vi "Lock Controls.vi"(8 "error in (no error)":errorcluster, 10 "Lock Controls?":bool, 11 "PXIe5105 in":refnum<class "PXIe5105.lvclass">) -> (0 "error out":errorcluster, 3 "PXIe5105 out":refnum<class "PXIe5105.lvclass">)   [LabVIEW 2018, in "PXIe5105.lvlib" / "PXIe5105.lvclass"]
doc: "This override method is used to lock/unlock user access to the oscilloscope front panel controls."
uses:
  PXIe5105.lvclass
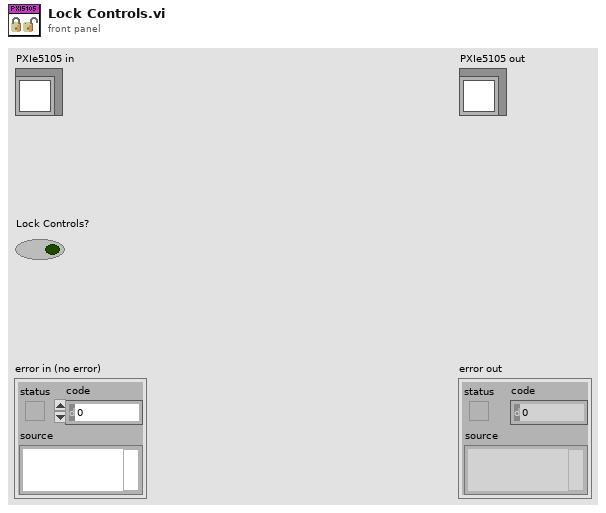
[diagram p1: front panel]
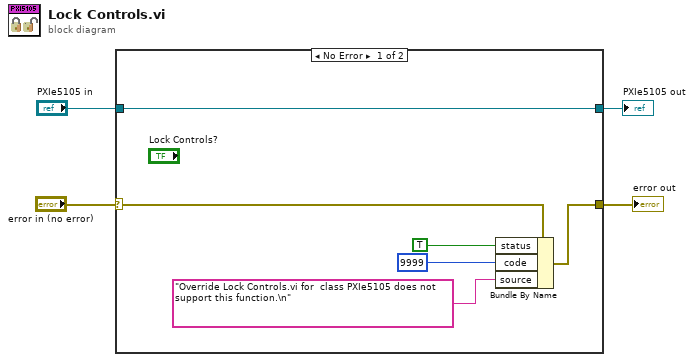
[diagram p0: block diagram]
diagram:
  n1 = case shown="No Error" "error in (no error)" {
    selector: "error in (no error)" -> [w7 w12]
    tunnel: [w6 w12] -> w3
    tunnel: [w5 w11] -> w2
    tunnel: "PXIe5105 in" -> [w5 w11]
    frame No Error {
      n2 = Bundle By Name(cluster=w7, "status"=TRUE, "code"=9999, "source"="Override Lock Controls.vi for  class PXIe5105 does not support this function.\n") -> (w6:errorcluster)
    }
    frame Error {
    }
  }
  "error out" <- w3
  "PXIe5105 out" <- w2
